vi "tcp_read_null.vi"(8 "error in (no error)":errorcluster, 9 "timeout ms (10000)":i32=10000, 11 "conn in":refnum<k5>) -> (0 "error out":errorcluster, 2 "data out":string, 3 "conn out":refnum<k5>)   [LabVIEW 2017, in "rethinkdb.lvlib"]
uses:
  rethinkdb.lvlib
  debug_action.ctl
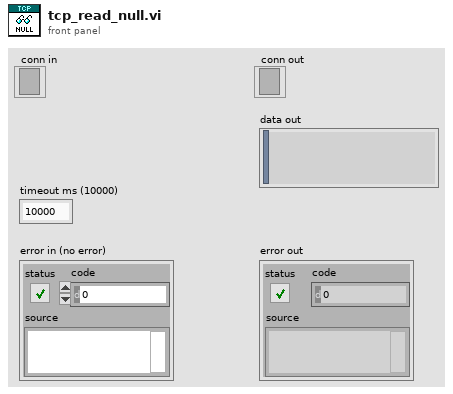
[diagram p1: front panel]
types:
  T1 = typedef "rethinkdb.lvlib/debug_action.ctl" = enum8{"get", "set_query", "set_response", "clear"}
  T2 = enum16{"Standard", "Buffered", "CRLF", "Immediate"}
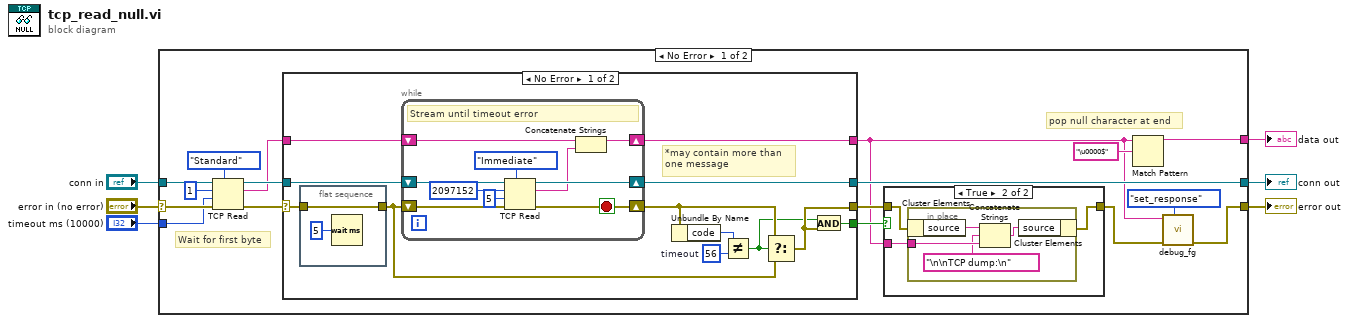
[diagram p0: block diagram]
diagram:
  n1 = case shown="No Error" "error in (no error)" {
    selector: "error in (no error)" -> [w22 w60]
    tunnel: "conn in" -> [w23 w59]
    tunnel: "timeout ms (10000)" -> [w21 _]
    tunnel: [w10 w60] -> w3
    tunnel: [w17 w59] -> w2
    tunnel: [w8 _] -> w1
    frame No Error {
      # "pop null character at end"
      # "Wait for first byte"
      n2 = TCP Read(connection ID=w23, bytes to read=1, error in (no error)=w22, 7:T2."Standard" ("mode (standard)"), 9:w21) -> (connection ID out=w16:refnum<k5>, data out=w15:string, error out=w18:errorcluster)
      n3 = case shown="No Error" w18 {
        selector: w18 -> [w35 w50]
        tunnel: [w26 w50] -> w14
        tunnel: [w33 w49] -> w17
        tunnel: w16 -> [w34 w49]
        tunnel: w15 -> [w32 w48]
        tunnel: [w31 w48] -> w7
        tunnel: [w24 _] -> w13
        frame No Error {
          w29 = 56  # timeout
          # "*may contain more than\none message"
          n4 = flat-sequence {
            tunnel: [w46] -> w27
            tunnel: w35 -> [w46]
            frame #0 {
              n5 = Wait (ms)(milliseconds to wait=u32 5) -> ()  [unwired: 1 out]
            }
          }
          n6 = while {
            shift-right: [w37] -> w28
            shift-left: w27 -> [w45]
            shift-right: [w43] -> w33
            shift-left: w34 -> [w44]
            shift-right: [w36] -> w31
            shift-left: w32 -> [w39]
            stop <- w37 stop-if-true
            # "Stream until timeout error"
            n7 = TCP Read(connection ID=w44, bytes to read=2097152, error in (no error)=w45, 7:T2."Immediate" ("mode (standard)"), 9:5 ("timeout ms (25000)")) -> (connection ID out=w43:refnum<k5>, data out=w38:string, error out=w37:errorcluster)
            n8 = Concatenate Strings(w39, w38) -> (w36:string)
          }
          n9 = Unbundle By Name(w28) -> ("code"=w30:i32)
          n10 = Not Equal?(x=w30, y=w29) -> (x != y?=w25:bool)
          n11 = Select(t=w28, s=w25, f=w27) -> (s? t:f=w26:errorcluster)
          n12 = And(x=w25, y=w26) -> (x .and. y?=w24:bool)
        }
        frame Error {
        }
      }
      n13 = case shown="True" w13 {
        tunnel: w7 -> [_ w54]
        tunnel: [w51 w53] -> w9
        tunnel: w14 -> [w51 w52]
        frame False {
        }
        frame True {
          n14 = in-place {
            in-place-border: w54 -> [w56]
            n15 = in-place-cluster #1(w52) -> ("source"=w58:string)
            n16 = Concatenate Strings(w58, "\n\nTCP dump:\n" ("format string"), w56) -> (w57:string)
            n17 = in-place-cluster #1("source"=w57) -> (w53:errorcluster)
          }
        }
      }
      n18 = Match Pattern(string=w7, regular expression="\u0000$") -> (before substring=w8:string)  [unwired: 1 in, 3 out]
      n19 = call "debug_fg.vi"("action"=debug_action."set_response", "error in (no error)"=w9, "data"=w7) -> ("error out"=w10:errorcluster)  [unwired: 7 in, 1 out]
    }
    frame Error {
    }
  }
  "error out" <- w3
  "conn out" <- w2
  "data out" <- w1
